vi "Make Cancelable Observer.vi"(8 "error in (no error)":errorcluster, 11 "Observer In":refnum<class "Observer.lvclass">) -> (0 "error out":errorcluster, 3 "CancelableObserver out":refnum<class "CancelableObserver.lvclass">)   [LabVIEW 2011, in "Messenging.lvlib" / "CancelableObserver.lvclass"]
uses:
  CancelableObserver.lvclass
  SendOnly/Observer.lvclass
  CancelableObserver.lvclass/CancelableObserver.ctl
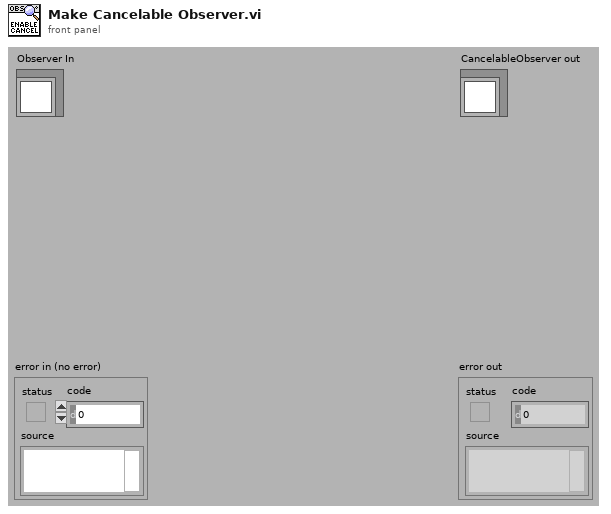
[diagram p1: front panel]
types:
  T1 = typedef "Semaphore RefNum" = refnum<k1>
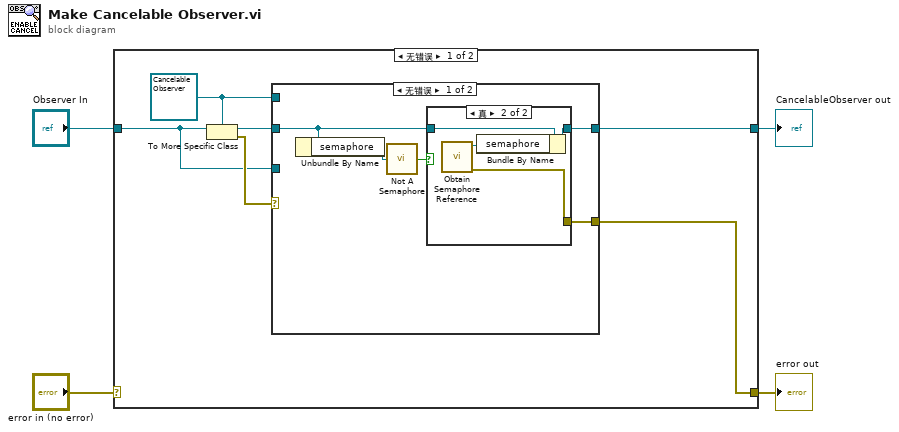
[diagram p0: block diagram]
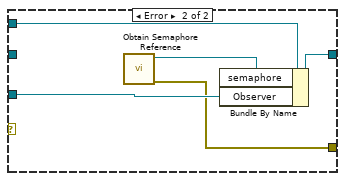
[diagram p3: hidden frame]
diagram:
  n1 = case shown="无错误" "error in (no error)" {
    selector: "error in (no error)" -> [_ w26]
    tunnel: [w9 w26] -> w3
    tunnel: [w10 _] -> w1
    tunnel: "Observer In" -> [w6 _]
    frame No Error {
      w5 = refnum<class "CancelableObserver.lvclass"> refnum ("Messenging.lvlib:CancelableObserver.lvclass")
      n2 = To More Specific Class(target class=w5, reference=w6) -> (specific class reference=w8:refnum<class "CancelableObserver.lvclass">, error out=w7:errorcluster)  [unwired: 1 in]
      n3 = case shown="无错误" w7 {
        tunnel: [w14 w24] -> w10
        tunnel: [w15 w21] -> w9
        tunnel: w8 -> [w13 _]
        tunnel: w6 -> [_ w22]
        tunnel: w5 -> [_ w25]
        frame No Error {
          n4 = Unbundle By Name(w13) -> ("semaphore"=w12:T1)
          n5 = call <vilib>:"Not A Semaphore.vi"("semaphore"=w12) -> ("not a semaphore"=w11:bool)
          n6 = case shown="真" w11 {
            tunnel: [_ w19] -> w15
            tunnel: [w16 w18] -> w14
            tunnel: w13 -> [w16 w17]
            frame False {
            }
            frame True {
              n7 = call <vilib>:"Obtain Semaphore Reference.vi"() -> ("error out"=w19:errorcluster, "semaphore"=w20:T1)  [unwired: 3 in, 3 out]
              n8 = Bundle By Name(cluster=w17, "semaphore"=w20) -> (w18:refnum<class "CancelableObserver.lvclass">)
            }
          }
        }
        frame Error {
          n9 = call <vilib>:"Obtain Semaphore Reference.vi"() -> ("error out"=w21:errorcluster, "semaphore"=w23:T1)  [unwired: 3 in, 3 out]
          n10 = Bundle By Name(cluster=w25, "semaphore"=w23, "Observer"=w22) -> (w24:refnum<class "CancelableObserver.lvclass">)
        }
      }
    }
    frame Error {
    }
  }
  "error out" <- w3
  "CancelableObserver out" <- w1
